vi "Build Engine Name.vi"(1 "Current Bus Number":i32) -> (0 "Engine Name":string)   [LabVIEW 2014, in "Initialization and IO Node Scripting.lvlib"]
uses:
  Initialization and IO Node Scripting.lvlib
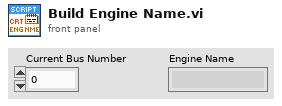
[diagram p1: front panel]
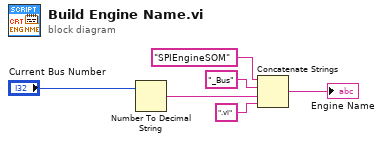
[diagram p0: block diagram]
diagram:
  n1 = Number To Decimal String(number="Current Bus Number") -> (decimal integer string=w2:string)  [unwired: 1 in]
  n2 = Concatenate Strings("SPIEngineSOM" ("string"), "_Bus" ("string"), w2, ".vi" ("string")) -> (→"Engine Name":string)
